vi "Fetch Trace.vi"(8 "error in (no error)":errorcluster, 9 "Timeout (10000 ms)":i32=10000, 10 "Trace Name (1: Trace 1)":u16(ring)=1 items=["Trace 1"=1, "Trace 2"=2, "Trace 3"=3, "Trace 4"=4, "Trace 5"=5, "Trace 6"=6, "LLINE 1"=7, "LLINE 2"=8], 11 "VISA resource name":refnum<visa-resource-name>) -> (0 "error out":errorcluster, 2 "Trace Array":dbl[](array[numeric]), 3 "VISA resource name out":refnum<visa-resource-name>, 5 "X Increment":dbl, 7 "Initial X":dbl)   [LabVIEW 2014, in "Agilent ESA PSA Series.lvlib"]
doc: "Returns the acquired trace and scaling information from the spectrum analyzer. The trace is from an acquisition that you initiate prior to calling this VI. You initiate an acquisition with the Initiate VI.\n\n<B>Note:</B> \n\nUse this VI only with other low-level VIs. The high-level VIs automatically incorporate this functionality. This VI does not check the instrument status."
uses:
  Agilent ESA PSA Series.lvlib
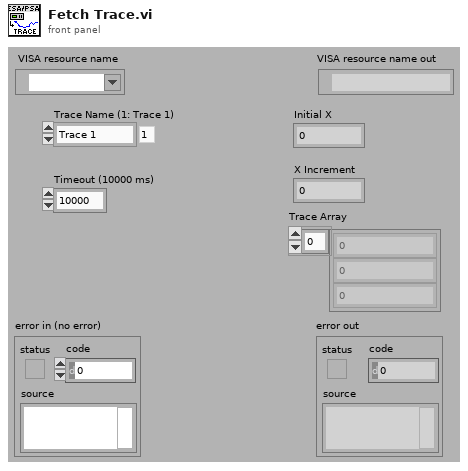
[diagram p1: front panel]
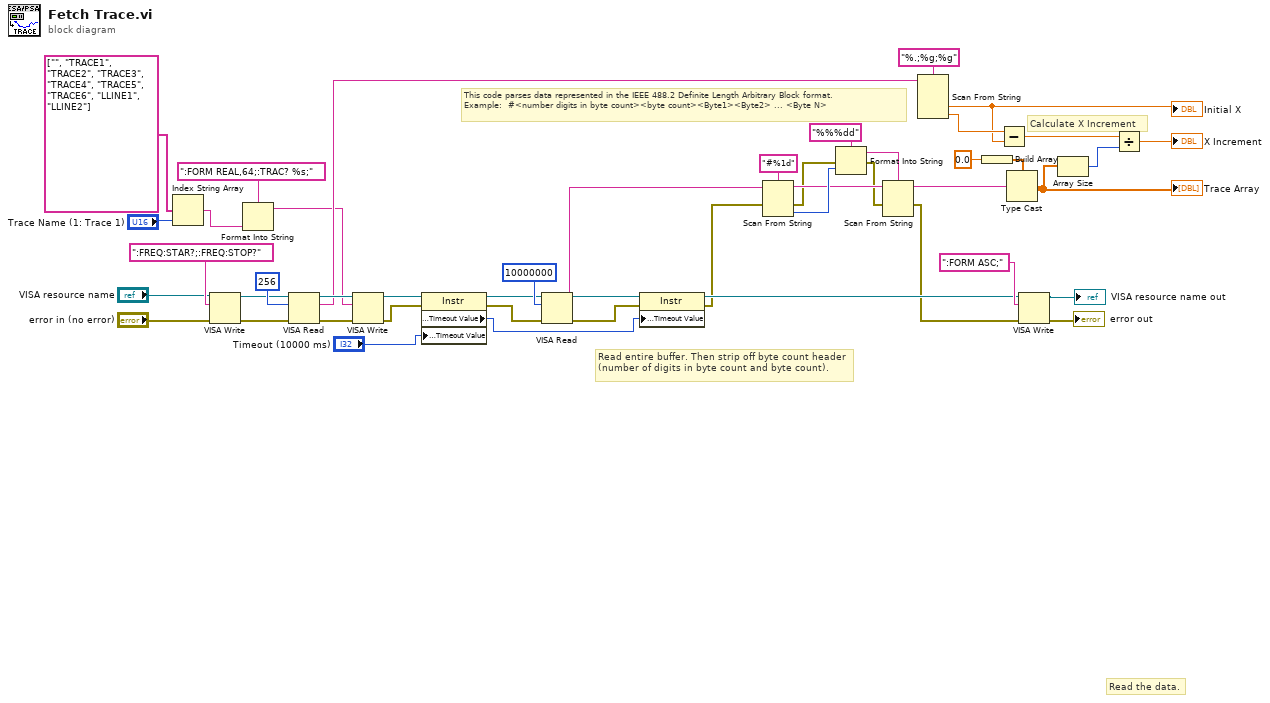
[diagram p0: block diagram]
diagram:
  # "Read entire buffer. Then strip off byte count header (number of digits in byte count and byte count)."
  # "This code parses data represented in the IEEE 488.2 Definite Length Arbitrary Block format.\nExample:  #<number digits in byte count><byte count><Byte1><Byte2> ... <Byte N>"
  # "Read the data."
  # "Calculate X Increment"
  n1 = Index String Array(1:"Trace Name (1: Trace 1)", 2:string[] ["", "TRACE1", "TRACE2", "TRACE3", "TRACE4", "TRACE5", "TRACE6", "LLINE1", "LLINE2"]) -> (0:w30:string)  [unwired: 1 in]
  n2 = VISA Write(VISA resource name="VISA resource name", write buffer=":FREQ:STAR?;:FREQ:STOP?", error in (no error)="error in (no error)") -> (VISA resource name out=w42:refnum<visa-resource-name>, error out=w39:errorcluster)  [unwired: 1 out]
  n3 = Format Into String(format string=":FORM REAL,64;:TRAC? %s;" ("Fetch Measurement"), w30) -> (resulting string=w29:string)  [unwired: 2 in, 1 out]
  n4 = VISA Read(VISA resource name=w42, byte count=u32 256, error in (no error)=w39) -> (VISA resource name out=w41:refnum<visa-resource-name>, read buffer=w37:string, error out=w40:errorcluster)  [unwired: 1 out]
  n5 = VISA Write(VISA resource name=w41, write buffer=w29, error in (no error)=w40) -> (VISA resource name out=w14:refnum<visa-resource-name>, error out=w13:errorcluster)  [unwired: 1 out]
  n6 = property on="Property Node" class="Instr"(reference=w14, error in=w13, "General Settings:Timeout Value"="Timeout (10000 ms)") -> (reference out=w12:refnum<visa-resource-name>, error out=w11:errorcluster, "General Settings:Timeout Value"=w1:u32)
  n7 = VISA Read(VISA resource name=w12, byte count=u32 10000000, error in (no error)=w11) -> (VISA resource name out=w8:refnum<visa-resource-name>, read buffer=w24:string, error out=w6:errorcluster)  [unwired: 1 out]
  n8 = property on="Property Node" class="Instr"(reference=w8, error in=w6, "General Settings:Timeout Value"=w1) -> (reference out=w7:refnum<visa-resource-name>, error out=w5:errorcluster)
  n9 = Scan From String(format string="#%1d", input string=w24, error in=w5) -> (remaining string=w21:string, error out=w4:errorcluster, output 1=w23:i32)  [unwired: 2 in, 1 out]
  n10 = Format Into String(format string="%%%dd", error in=w4, w23) -> (resulting string=w22:string, error out=w3:errorcluster)  [unwired: 1 in]
  n11 = Scan From String(format string=w22, input string=w21, error in=w3) -> (remaining string=w18:string, error out=w2:errorcluster)  [unwired: 3 in, 1 out]
  n12 = Scan From String(format string="%.;%g;%g", input string=w37) -> (output 1=w35:dbl, output 2=w36:dbl)  [unwired: 4 in, 3 out]
  "Initial X" <- w35
  n13 = Build Array(0.0) -> (w28:dbl[])
  n14 = Subtract(x=w36, y=w35) -> (x-y=w45:dbl)
  n15 = Type Cast(type=w28, x=w18) -> (*(type *) &x=w27:dbl[])
  "Trace Array" <- w27
  n16 = VISA Write(VISA resource name=w7, write buffer=":FORM ASC;" ("Fetch Measurement"), error in (no error)=w2) -> (VISA resource name out=→"VISA resource name out":refnum<visa-resource-name>, error out=→"error out":errorcluster)  [unwired: 1 out]
  n17 = Array Size(array=w27) -> (size(s)=w44:i32)
  n18 = Divide(x=w45, y=w44) -> (x/y=→"X Increment":dbl)
